vi "TSLIN_Write.vi"(8 "错误输入（无错误）":errorcluster, 9 "TLIBLIN":T2, 11 "路径输入":path) -> (0 "错误输出":errorcluster, 2 "result":i32, 3 "路径输出":path)   [LabVIEW 2019]
uses:
  Typedef/TLibLIN.ctl
panel:
  in  "ADataArray":T1
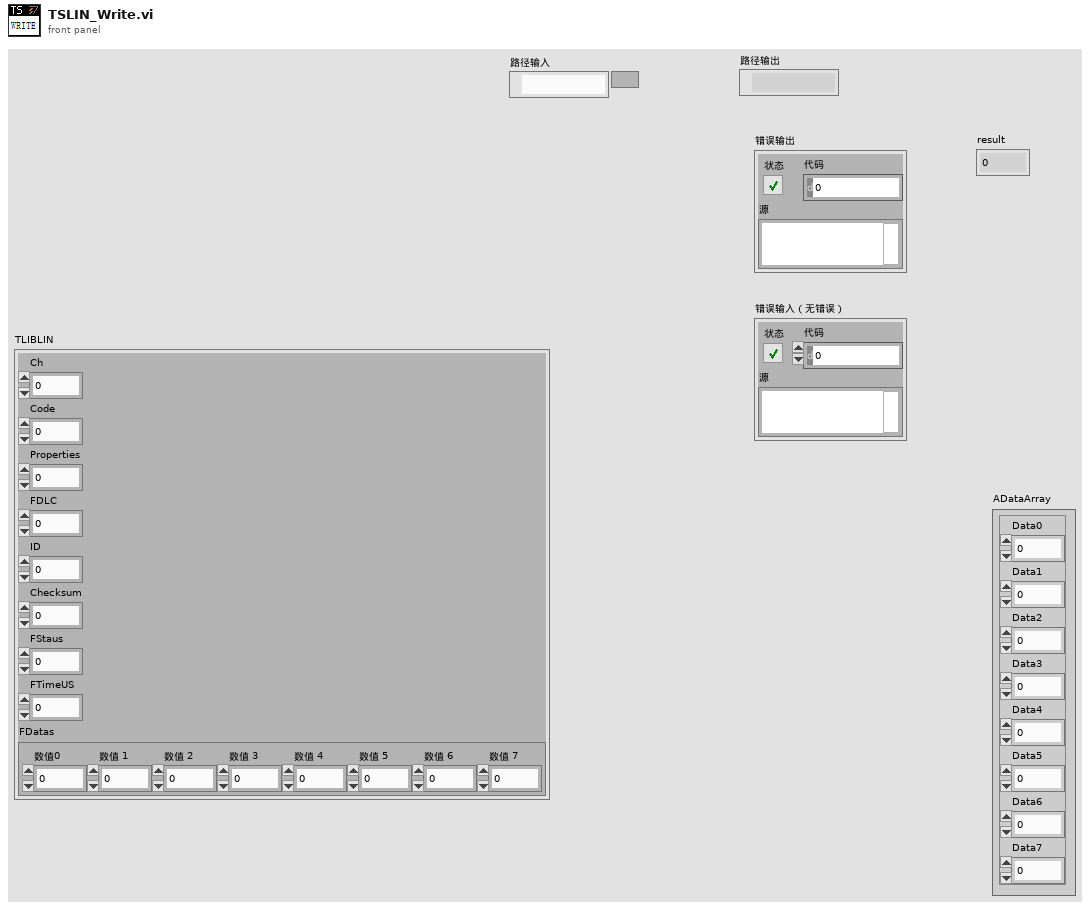
[diagram p1: front panel]
types:
  T1 = cluster{"Data0":u8, "Data1":u8, "Data2":u8, "Data3":u8, "Data4":u8, "Data5":u8, "Data6":u8, "Data7":u8}
  T2 = typedef "TLibLIN.ctl" = cluster{"Ch":u8, "Code":u8, "Properties":u8, "FDLC":u8, "ID":u8, "Checksum":u8, "FStaus":u8, "FTimeUS":u64, "FDatas":cluster{"数值0":u8, "数值 1":u8, "数值 2":u8, "数值 3":u8, "数值 4":u8, "数值 5":u8, "数值 6":u8, "数值 7":u8}}
  T3 = cluster{"数值0":u8, "数值 1":u8, "数值 2":u8, "数值 3":u8, "数值 4":u8, "数值 5":u8, "数值 6":u8, "数值 7":u8}
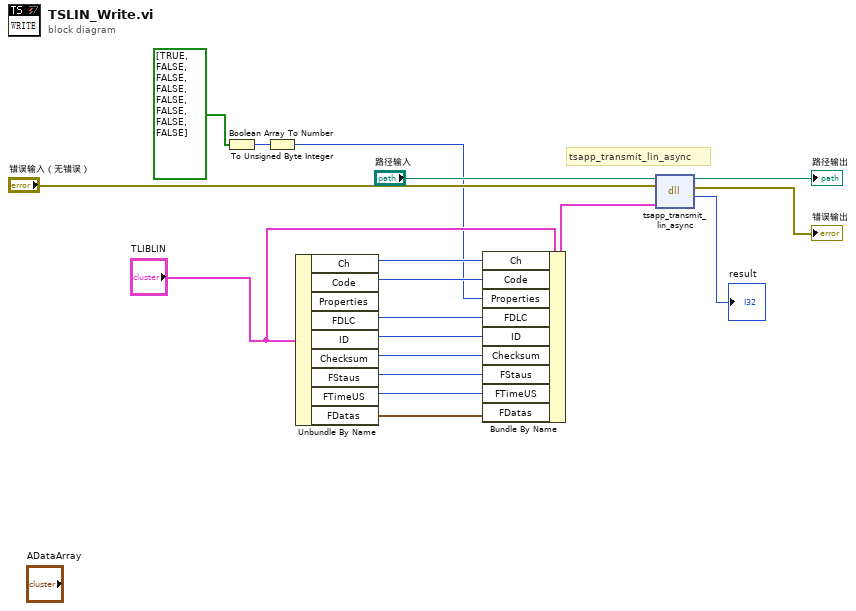
[diagram p0: block diagram]
diagram:
  # "tsapp_transmit_lin_async"
  n1 = Boolean Array To Number(Boolean array=bool[] [TRUE, FALSE, FALSE, FALSE, FALSE, FALSE, FALSE, FALSE]) -> (number=w13:u32)
  n2 = To Unsigned Byte Integer(number=w13) -> (unsigned 8bit integer=w8:u8)
  n3 = Unbundle By Name("TLIBLIN") -> ("Ch"=w11:u8, "Code"=w10:u8, "FDLC"=w7:u8, "ID"=w6:u8, "Checksum"=w5:u8, "FStaus"=w4:u8, "FTimeUS"=w3:u64, "FDatas"=w1:T3)  [unwired: 1 out]
  n4 = Bundle By Name(cluster="TLIBLIN", "Ch"=w11, "Code"=w10, "Properties"=w8, "FDLC"=w7, "ID"=w6, "Checksum"=w5, "FStaus"=w4, "FTimeUS"=w3, "FDatas"=w1) -> (w2:T2)
  n5 = dll-call lib="PTH2@abs EDemo同星TSCAN_V1.4_20220301ConfigTSMaster.dll" fn="tsapp_transmit_lin_async"(path in="路径输入", error in="错误输入（无错误）", "LINDATA"=w2) -> (path out=→"路径输出":path, error out=→"错误输出":errorcluster, "tsapp_transmit_can_async"=→"result":i32)  [unwired: 2 in]
